vi "Wire Two Terminals.vi"(8 "error in (no error)":errorcluster, 10 "Sink Terminal in":refnum<vi>, 11 "Source Terminal":refnum<vi>) -> (0 "error out":errorcluster, 3 "Source Terminal out":refnum<vi>)   [LabVIEW 2019, in "gRPC Template Creation Utility.lvlib"]
uses:
  gRPC Template Creation Utility.lvlib
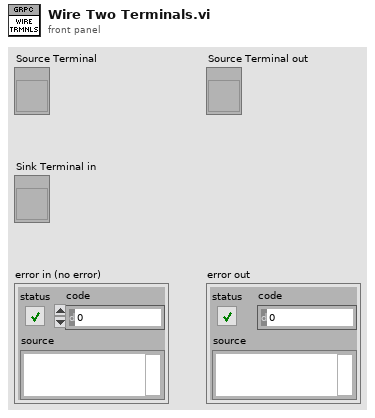
[diagram p1: front panel]
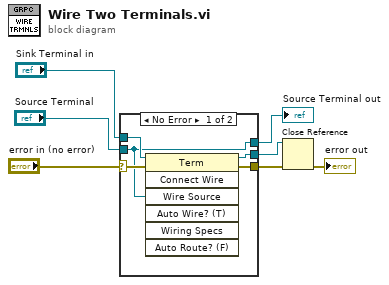
[diagram p0: block diagram]
diagram:
  n1 = case shown="No Error" "error in (no error)" {
    selector: "error in (no error)" -> [w9 w14]
    tunnel: "Source Terminal" -> [w8 w13]
    tunnel: [w12 w14] -> w3
    tunnel: [w11 w15] -> w1
    tunnel: "Sink Terminal in" -> [w10 w15]
    tunnel: [w8 w13] -> w4
    frame No Error {
      n2 = invoke class="Term" method="Connect Wire"(reference=w10, error in=w9, "Wire Source"=w8) -> (reference out=w11:refnum<vi>, error out=w12:errorcluster)  [unwired: 4 in, 5 out]
    }
    frame Error {
    }
  }
  "Source Terminal out" <- w4
  n3 = Close Reference(reference=w1, error in (no error)=w3) -> (error out=→"error out":errorcluster)
